vi "Analysator Liste komplettieren.vi"(11 "AnalysatorDefinition Array in":T2[](array[typedef])) -> (1 "Analysatoren Strings And Values[]":T1(array[cluster]), 2 "Analysator String Array out":string[][](array[string]), 3 "AnalysatorDefinition Array out":T2[](array[typedef]))   [LabVIEW 2020, in "System Einstellungen V2.lvlib"]
uses:
  System Einstellungen V2.lvlib
  AnalysatorDefinition.ctl
  Analysator Definition/FGV Analysator Definition Aktionen.ctl
  Analysator Definition/Analysator Definition.lvlib
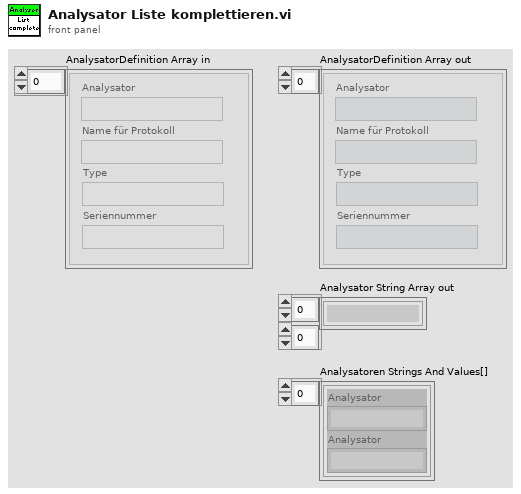
[diagram p1: front panel]
types:
  T1 = cluster{"Analysator":string, "Analysator":string}[]
  T2 = typedef "System Einstellungen V2.lvlib/AnalysatorDefinition.ctl" = cluster{"Analysator":string, "Name für Protokoll":string, "Type":string, "Seriennummer":string}
  T3 = typedef "Analysator Definition.lvlib/FGV Analysator Definition Aktionen.ctl" = enum16{"lesen", "MB setzen", "MB KAL setzen", "laden"}
  T4 = cluster{"Analysator":string, "Analysator":string}
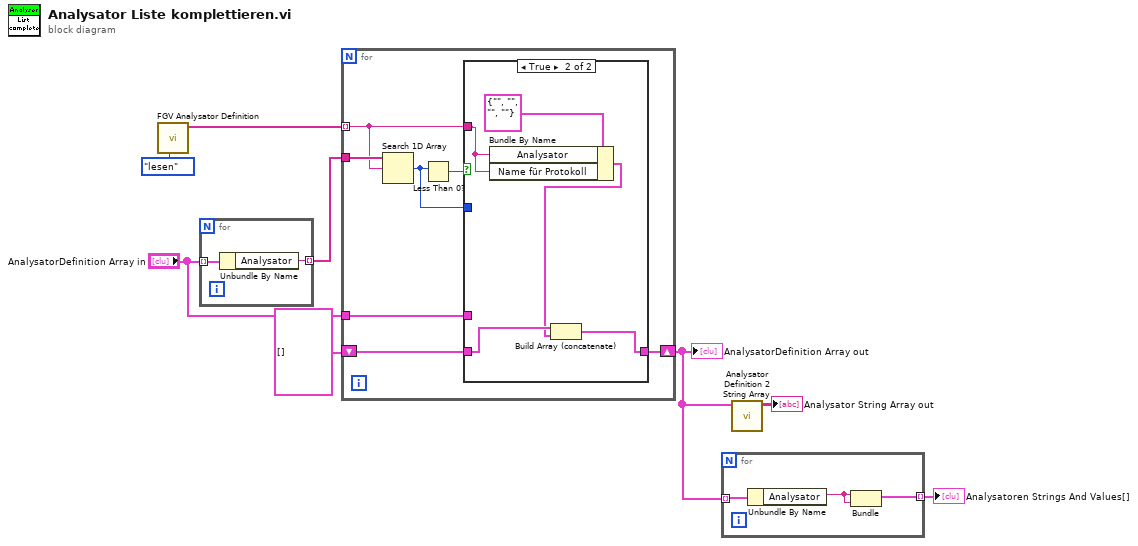
[diagram p0: block diagram]
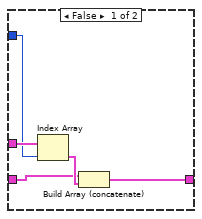
[diagram p2: hidden frame]
diagram:
  n1 = call "FGV Analysator Definition.vi"("Aktionen"=FGV_Analysator_Definition_Aktionen."lesen") -> ("Analysatoren"=w7:string[])  [unwired: 6 in, 4 out]
  n2 = for {
    tunnel: "AnalysatorDefinition Array in" -> [w10] mode=indexing
    tunnel: [w9] -> w6 mode=indexing
    n3 = Unbundle By Name(w10) -> ("Analysator"=w9:string)
  }
  n4 = for {
    tunnel: w7 -> [w11] mode=indexing
    tunnel: w6 -> [w17]
    tunnel: "AnalysatorDefinition Array in" -> [w14]
    shift-right: [w13] -> w2
    shift-left: T2[] [] -> [w12]
    n5 = Search 1D Array(1D array=w17, element=w11) -> (index of element=w15:i32)  [unwired: 1 in]
    n6 = Less Than 0?(x=w15) -> (x < 0?=w16:bool)
    n7 = case shown="True" w16 {
      tunnel: w15 -> [w18 _]
      tunnel: w14 -> [w22 _]
      tunnel: [w20 w24] -> w13
      tunnel: w12 -> [w19 w25]
      tunnel: w11 -> [_ w26]
      frame False {
        n8 = Index Array(array=w22, index=w18) -> (element=w21:T2)
        n9 = Build Array (concatenate)(w19, w21) -> (w20:T2[])
      }
      frame True {
        n10 = Bundle By Name(cluster=T2 {"Analysator"="", "Name für Protokoll"="", "Type"="", "Seriennummer"=""} ("AnalysatorDefinition"), "Analysator"=w26, "Name für Protokoll"=w26) -> (w23:T2)
        n11 = Build Array (concatenate)(w25, w23) -> (w24:T2[])
      }
    }
  }
  "AnalysatorDefinition Array out" <- w2
  n12 = for {
    tunnel: w2 -> [w30] mode=indexing
    tunnel: [w29] -> w1 mode=indexing
    n13 = Unbundle By Name(w30) -> ("Analysator"=w28:string)
    n14 = Bundle("Analysator"=w28, "Analysator"=w28) -> (w29:T4)  [unwired: 1 in]
  }
  "Analysatoren Strings And Values[]" <- w1
  n15 = call "Analysator Definition 2 String Array.vi"("AnalysatorDefinition Array in"=w2) -> ("Analysator String Array"=→"Analysator String Array out":string[][])  [unwired: 10 in]
